vi "Get Generated gRPC API Path.vi"(8 "error in":errorcluster, 10 "proto file name":string="data_store_service.proto", 11 "source proto directory":path=path "C:/dev/ASW/Source/Protos") -> (0 "error out":errorcluster, 2 "proto file path":path, 3 "api path":path)   [LabVIEW 2024, in "gRPC Client Generation.lvlib"]
uses:
  gRPC Client Generation.lvlib
  <vilib>/Utility/error.llb/Error Cluster From Error Code.vi
  <vilib>/ErrorRing/Error Ring.xnode
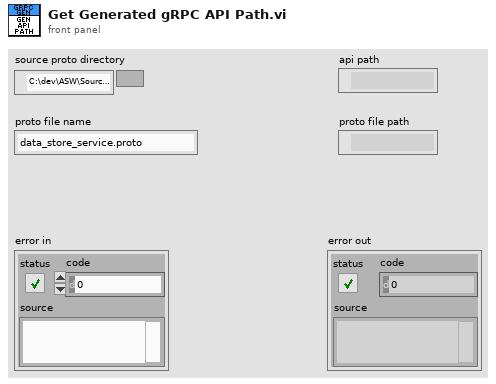
[diagram p1: front panel]
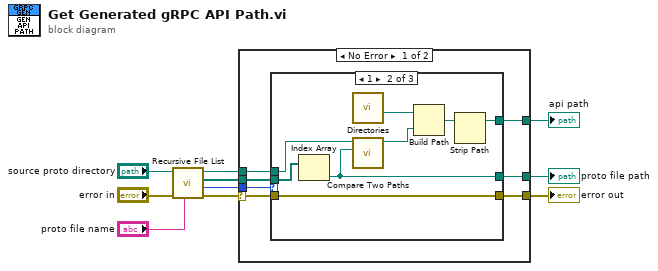
[diagram p0: block diagram]
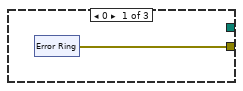
[diagram p2: hidden frame]
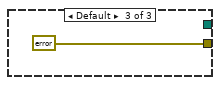
[diagram p3: hidden frame]
diagram:
  n1 = call <vilib>:"Recursive File List.vi"("pattern"="proto file name", "error in (no error)"="error in", "Folder Path"="source proto directory") -> ("error out"=w7:errorcluster, "Number of Files"=w6:i32, "All Files in Dir"=w5:path[], "dup Folder Path"=w4:path)  [unwired: 4 in, 1 out]
  n2 = case shown="No Error" w7 {
    selector: w7 -> [w14 w32]
    tunnel: w6 -> [w17 _]
    tunnel: w5 -> [w16 _]
    tunnel: w4 -> [w15 _]
    tunnel: [w13 w32] -> w3
    tunnel: [w12 _] -> w2
    tunnel: [w11 _] -> w1
    frame No Error {
      n3 = case shown="1" w17 {
        tunnel: [w18 w26 errorcluster {"status"=TRUE, "code"=5001, "source"="Found multiple proto files with provided name."} ("error constant")] -> w13
        tunnel: w16 -> [_ w30 _]
        tunnel: w15 -> [_ w29 _]
        tunnel: w14 -> [_ w26 _]
        tunnel: [_ w25 _] -> w12
        tunnel: [_ w23 _] -> w11
        frame 0 {
          n4 = xnode "Error Ring"() -> ("error out"=w18:errorcluster)
        }
        frame 1 {
          n5 = Index Array(array=w30) -> (element=w23:path)  [unwired: 1 in]
          n6 = call "Directories.vi"() -> ("generated apis"=w28:path)  [unwired: 9 in, 2 out]
          n7 = call <vilib>:"Compare Two Paths.vi"("Path 2"=w23, "Path 1"=w29) -> ("Relative Path from 1 to 2"=w27:path)  [unwired: 6 in, 3 out]
          n8 = Build Path(base path=w28, name or relative path=w27) -> (appended path=w24:path)
          n9 = Strip Path(path=w24) -> (stripped path=w25:path)  [unwired: 1 out]
        }
        frame Default {
        }
      }
    }
    frame Error {
    }
  }
  "error out" <- w3
  "api path" <- w2
  "proto file path" <- w1
